vi "Write reading array.vi"(8 "error in (no error)":errorcluster, 10 "reading array":dbl[](array[numeric]) format="%^.2e", 11 "CS++DMM in":refnum<class "CS++DMM.lvclass">) -> (0 "error out":errorcluster, 3 "CS++DMM out":refnum<class "CS++DMM.lvclass">)   [LabVIEW 2013, in "CS++DMM.lvlib" / "CS++DMM.lvclass"]
doc: "Write measured values."
uses:
  CS++DMM.lvclass
  CS++DMM.lvclass/CS++DMM.ctl
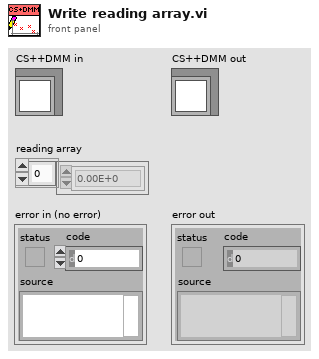
[diagram p1: front panel]
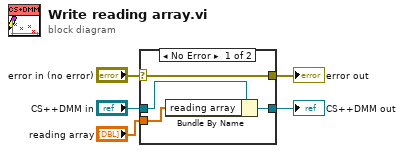
[diagram p0: block diagram]
diagram:
  n1 = case shown="No Error" "error in (no error)" {
    selector: "error in (no error)" -> [w9 w10]
    tunnel: [w9 w10] -> w4
    tunnel: [w7 w11] -> w2
    tunnel: "CS++DMM in" -> [w8 w11]
    tunnel: "reading array" -> [w6 _]
    frame No Error {
      n2 = Bundle By Name(cluster=w8, "reading array"=w6) -> (w7:refnum<class "CS++DMM.lvclass">)
    }
    frame Error {
    }
  }
  "error out" <- w4
  "CS++DMM out" <- w2
